vi "Read Outputs to system.vi"(8 "error in":errorcluster, 11 "Conversion runtime in":refnum<class "Conversion runtime.lvclass">) -> (0 "error out":errorcluster, 2 "Outputs to system":T1, 3 "Conversion runtime out":refnum<class "Conversion runtime.lvclass">)   [LabVIEW 2017, in "Conversion runtime.lvclass"]
uses:
  Conversion runtime.lvclass
  configuration/output data indices.ctl
  Conversion runtime.lvclass/Conversion runtime.ctl
  configuration/Conversion configuration.lvclass
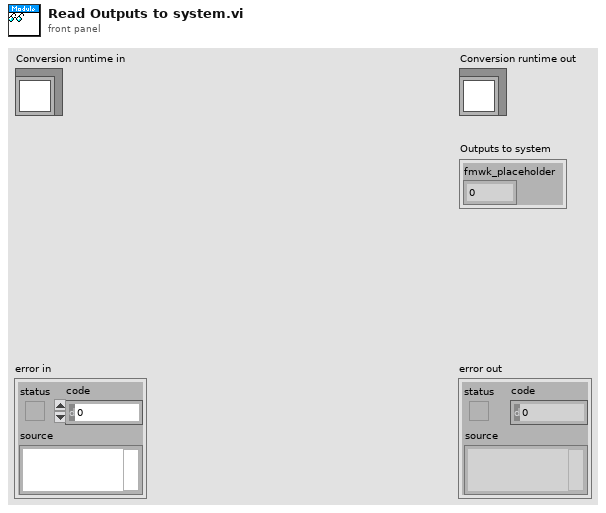
[diagram p1: front panel]
types:
  T1 = typedef "Conversion configuration.lvclass/output data indices.ctl" = cluster{"fmwk_placeholder":i32}
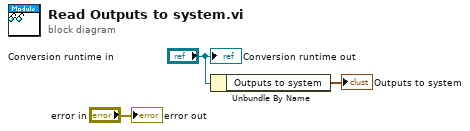
[diagram p0: block diagram]
diagram:
  n1 = Unbundle By Name("Conversion runtime in") -> ("Outputs to system"=→"Outputs to system":T1)
  "error out" <- "error in"
  "Conversion runtime out" <- "Conversion runtime in"
